vi "Display.vi"(8 "Error In":errorcluster, 11 "reference in":refnum<class "ProxyImage.lvclass">) -> (0 "Error Out":errorcluster, 3 "reference out":refnum<class "ProxyImage.lvclass">)   [LabVIEW 2020, in "ProxyImage.lvclass"]
uses:
  ProxyImage.lvclass
  RealImage_class/RealImage.lvclass
  <vilib>/addons/GOOPUtility/GOOPUtility.lvlib
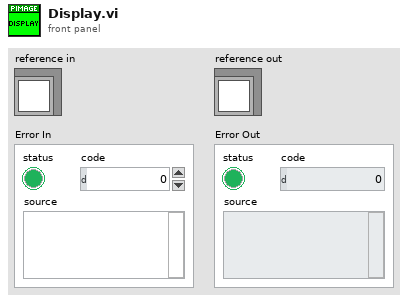
[diagram p1: front panel]
types:
  T1 = typedef "ProxyImage.lvclass/ObjectAttributes.ctl" = cluster{"_realImage":refnum<class "RealImage.lvclass">, "_fileName":string}
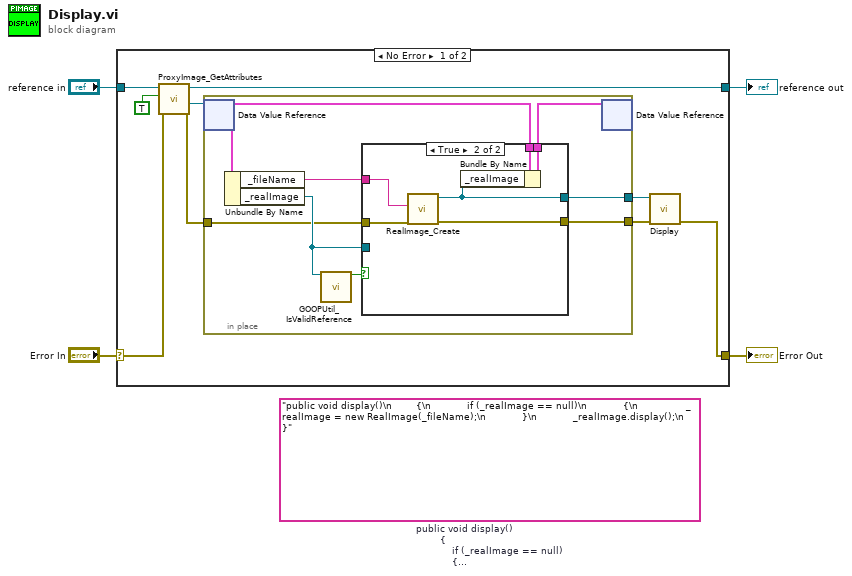
[diagram p0: block diagram]
diagram:
  (unwired) "public void display()\n        {\n            if (_realImage == null)\n            {\n                _realImage = new RealImage(_fileName);\n            }\n            _realImage.display();\n        }"  # public void display()         {             if (_realImage == null)             {                 _realImage = new RealImage(_fileName);             }             _realImage.display();         }
  n1 = case shown="No Error" "Error In" {
    selector: "Error In" -> [w12 w32]
    tunnel: [w6 w32] -> w3
    tunnel: [w11 w31] -> w1
    tunnel: "reference in" -> [w13 w31]
    frame No Error {
      n2 = call "ProxyImage_GetAttributes.vi"("error in (no error)"=w12, "OnlyGetDvrReference(False)"=TRUE, "reference in"=w13) -> ("error out"=w8:errorcluster, "DataRef"=w10:refnum<data-value>, "reference out"=w11:refnum<class "ProxyImage.lvclass">)  [unwired: 5 in, 1 out]
      n3 = in-place {
        in-place-border: w8 -> [w14]
        in-place-border: [w17] -> w7
        in-place-border: [w15] -> w5
        n4 = in-place-dvr #1(w10) -> (w20:T1)  [unwired: 1 out]
        n5 = Unbundle By Name(w20) -> ("_fileName"=w18:string, "_realImage"=w16:refnum<class "RealImage.lvclass">)
        n6 = call <vilib>:"GOOPUtil_IsValidReference.vi"("LabVIEW Object"=w16) -> ("Not a refnum?"=w19:bool)  [unwired: 16 in, 2 out]
        n7 = case shown="True" w19 {
          tunnel: [w23 w30] -> w21
          tunnel: w20 -> [w23 w29]
          tunnel: w14 -> [w24 w28]
          tunnel: w18 -> [_ w27]
          tunnel: [w24 w26] -> w17
          tunnel: w16 -> [w22 _]
          tunnel: [w22 w25] -> w15
          frame False {
          }
          frame True {
            n8 = call "RealImage_Create.vi"("Error In"=w28, "FileName"=w27) -> ("Error Out"=w26:errorcluster, "reference out"=w25:refnum<class "RealImage.lvclass">)  [unwired: 8 in]
            n9 = Bundle By Name(cluster=w29, "_realImage"=w25) -> (w30:T1)
          }
        }
        n10 = in-place-dvr #1(w21) -> ()  [unwired: 2 out]
      }
      n11 = call-dynamic "Display.vi"("Error In"=w7, "reference in"=w5) -> ("Error Out"=w6:errorcluster)  [unwired: 8 in, 1 out]
    }
    frame Error {
    }
  }
  "Error Out" <- w3
  "reference out" <- w1
